vi "Ball-Detect(Vision).vi"(8 "error in (no error)":errorcluster, 11 "Image Size":T5=enum."320x240") -> ()   [LabVIEW 2019]
uses:
  <vilib>/Rock Robotics/WPI/Camera/WPI_CameraImageSize.ctl
  vision/Camera Types.ctl
  <vilib>/Rock Robotics/WPI/Camera/WPI_CameraWhite Balance Values.ctl
  <vilib>/Rock Robotics/WPI/Camera/WPI_CameraFrameRate.ctl
  Robot Global Data.vi
  <vilib>/Rock Robotics/WPI/Camera/WPI_CameraExposure Values.ctl
  <vilib>/vision/NI_Vision_Development_Module.lvlib
panel:
  out "Disqualified":i32
  in  "Details":bool
  out "Results":T1(array[cluster]) {"Normalized Center"."x" format="%#_2g"; "Normalized Center"."y" format="%#_2g"; "Overall Score" format="%#_2g"; "Distance (ft)" format="%#_3g"; "Area Score" format="%#_2g"; "Moment Score" format="%#_2g"; "Aspect Score" format="%#_2g"}
  in  "Size Limit %":dbl=0.1 min=0.0 max=100.0 step=0.01 format="%#_13g"
  in  "Color Mode":u16(ring)=2 items=["RGB", "HSL", "HSV", "HSI"]
  in  "Particle Count LImit":i32=5
  in  "Score Threshold %":dbl=75.0
  in  "Std Devs for Calibration":cluster{"H":dbl, "S":dbl, "V":dbl}={"H"=4.0, "S"=8.0, "V"=8.0}
  in  "Camera Type (for distance)":T2=enum."MS HD3000 square"
  in  "Annotate":bool=TRUE
  out "Qualified":i32
  in  "Color Range":T3={"Hue"={24.535868437582977, 35.591417062105585}, "Sat"={188.21428571428572, 255.0}, "Val"={118.39285714285714, 255.0}} {"Hue" scale=0.0..255.0 scale format="%#_3g"}
  out "Mask":T4(plugin-control)
  out "Original Image":T4(plugin-control)
  out "Instructions:":string="Connect a USB or IP camera to your roboRIO. If using a ring light and retroreflective tape, use Camera Settings outside the loop create a dark image with bright and colorful stripes. If used wihtout a ring light, brighten the images so that stripes are visible.\n\nLED Color can encoded as HSL or related color modes. Calibrate to the same color as the strips being reflected to the camera. Unlike the desktop example, this LED color must be set by hand. You can also put the calibration on the dashboard and send the LED Color to the RT code using Network Tables.\n\nThe Display buttons affects whether images are displayed on the panel. It takes quite a bit of CPU  to compress and transmit the images for display.\n\nAdjust Score Cutoff to make the code more or less picky. If the color is not very unique, you may need to increase the number of particles considered. The diagram uses a Size Limit to ignore colored things that are too small. You may need to adjust it if you are targetting from far away.\n\nResults give you the distance to the target, the center and box in a normalized (-1 to 1) and pixel coordinates.\n\nBe sure to read about setting camera exposure and brightness to help simplify your image and acquire color saturated images.\n\nThere are lots of comments on the diagram to explain the code."
  out "loop ms":u32
  # "Scores"
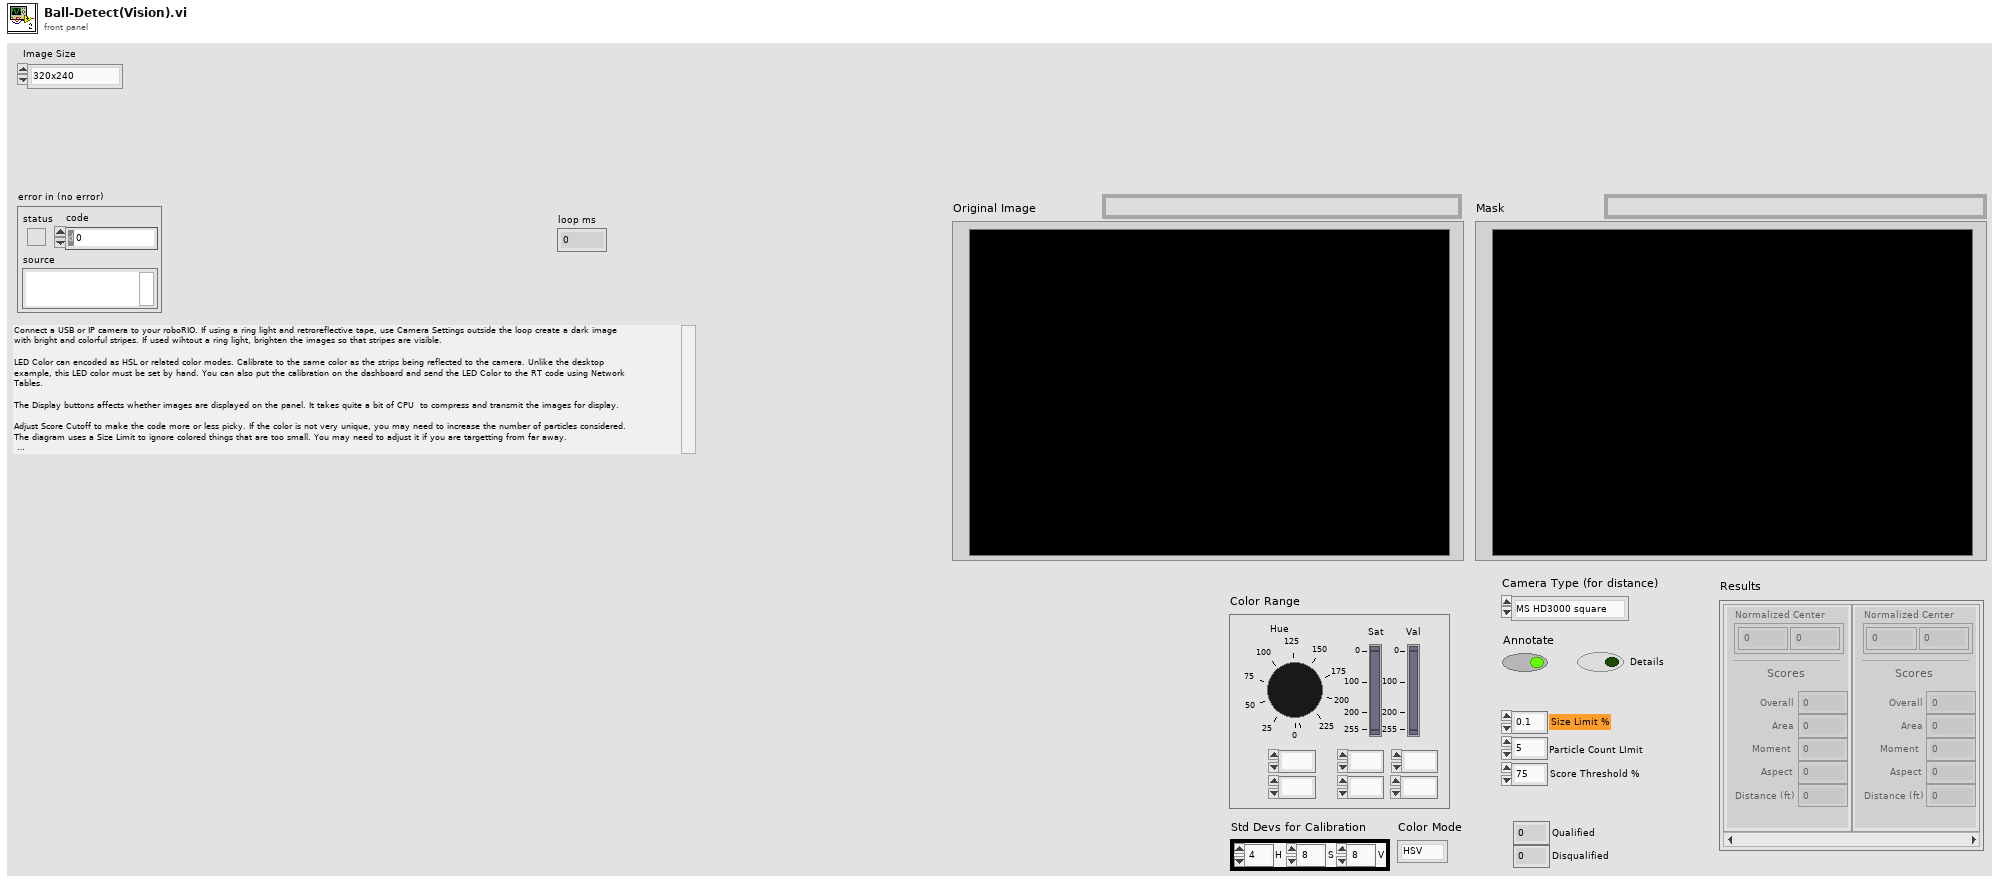
[diagram p1: front panel]
types:
  T1 = cluster{"diameter points":cluster{"first point":cluster{"x":dbl, "y":dbl}, "projected point":cluster{"x":dbl, "y":dbl}}, "Normalized Center":cluster{"x":dbl, "y":dbl}, "Overall Score":dbl, "Area Score":dbl, "Moment Score":dbl, "Aspect Score":dbl, "Distance (ft)":dbl, "Upper Goal":bool}[]
  T2 = typedef "Camera Types.ctl" = enum16{"206", "1011", "1013", "MS HD3000 square", "MS HD3000 640x480"}
  T3 = cluster{"Hue":cluster{dbl, dbl}, "Sat":cluster{dbl, dbl}, "Val":cluster{dbl, dbl}}
  T4 = typedef "IMAQ Image.ctl" = refnum<image>
  T5 = typedef "WPI_CameraImageSize.ctl" = enum16{"640x480", "320x240", "160x120", "Custom"}
  T6 = typedef "Particle Parameters" = i32
  T7 = typedef "WPI_CameraFrameRate.ctl" = u32
  T8 = typedef "WPI_CameraWhite Balance Values.ctl" = enum16{"Auto", "Fixed indoor", "Fixed outdoor 1", "Fixed outdoor 2", "Fixed fluorescent 1", "Fixed fluorescent 2", "Hold current", "Custom"}
  T9 = typedef "Image Type" = u32
  T10 = typedef "WPI_CameraDevRef.ctl" = cluster{"Camera Address":string, "CameraStatus":errorcluster}
  T11 = typedef "WPI_CameraExposure Values.ctl" = enum16{"Auto", "Flicker-free 50 Hz", "Flicker-free 60 Hz", "Hold current", "Custom"}
  T12 = cluster{cluster{dbl, dbl}, cluster{dbl, dbl}, cluster{dbl, dbl}}
  T13 = cluster{"remainder":i32, "size":bool, "count":bool}
  T14 = typedef "Target Fields.ctl" = cluster{"diameter points":cluster{"first point":cluster{"x":dbl, "y":dbl}, "projected point":cluster{"x":dbl, "y":dbl}}, "normalized center":cluster{"x":dbl, "y":dbl}, "Overall Score":dbl, "Area Score":dbl, "Moment Score":dbl, "Aspect Score":dbl, "Distance (ft)":dbl, "Upper Goal":bool}
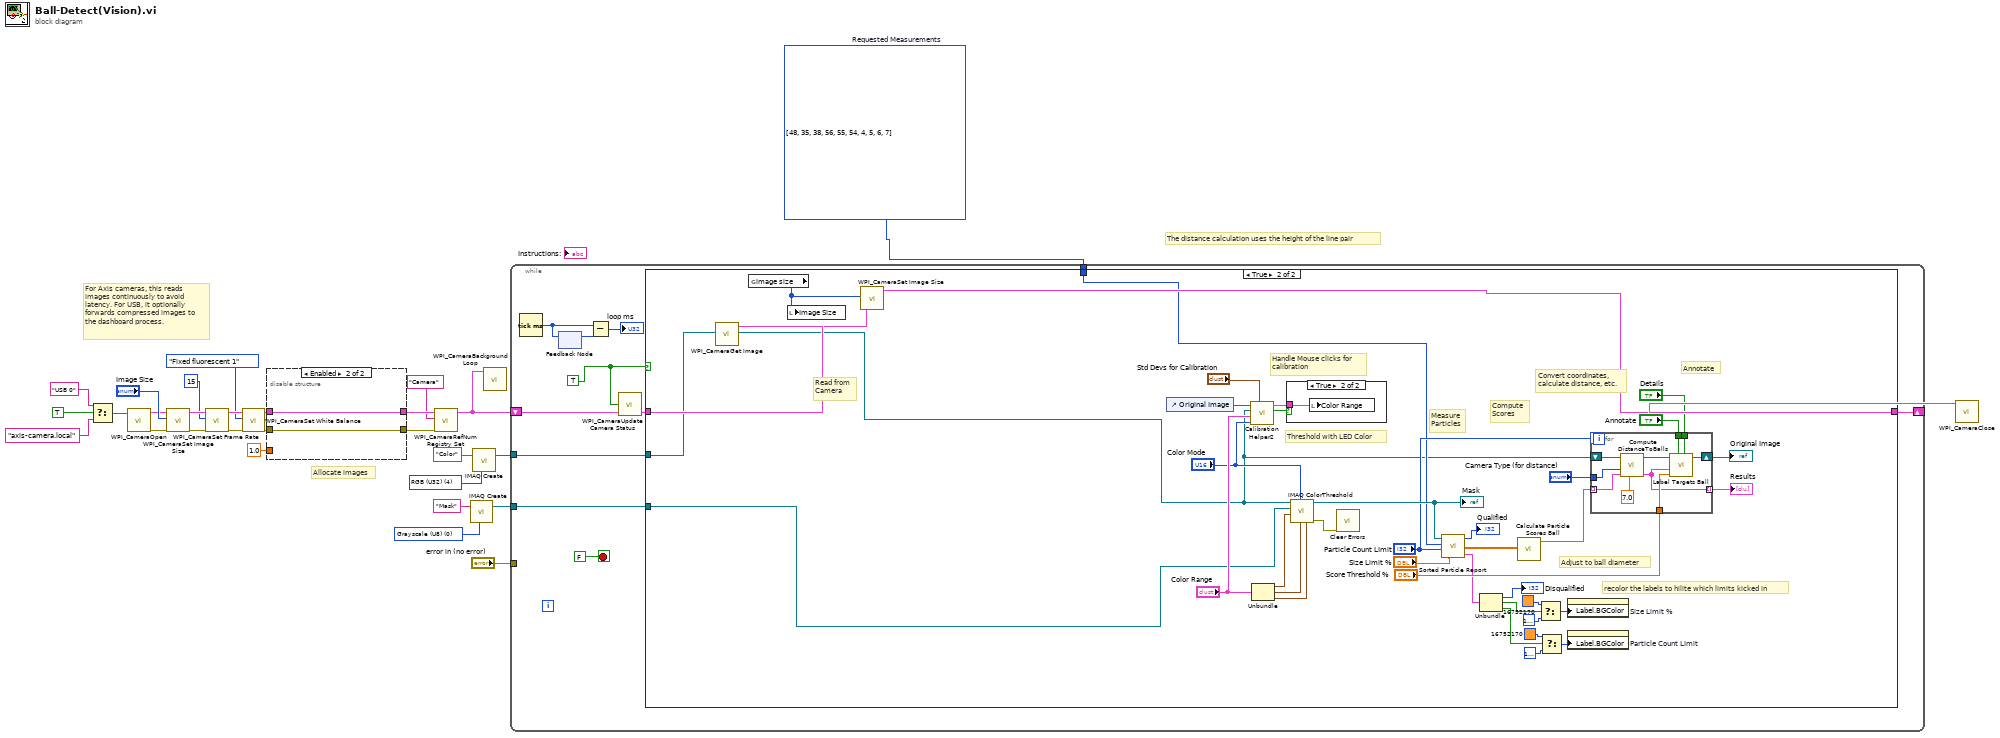
[diagram p0: block diagram]
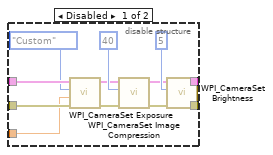
[diagram p2: hidden frame]
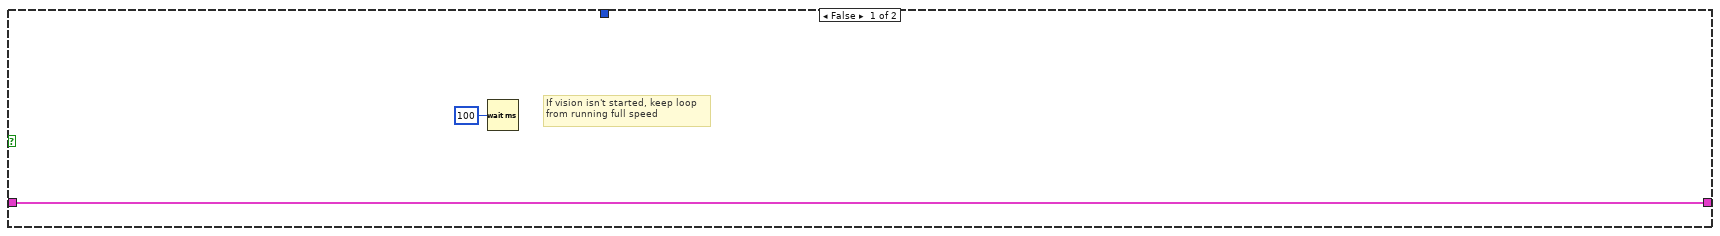
[diagram p3: hidden frame]
diagram:
  w1 = T6[] [48, 35, 38, 56, 55, 54, 4, 5, 6, 7] items=["Center of Mass X", "Center of Mass Y", "First Pixel X", "First Pixel Y", "Bounding Rect Left", "Bounding Rect Top", "Bounding Rect Right", "Bounding Rect Bottom", "Max Feret Diameter Start X", "Max Feret Diameter Start Y", "Max Feret Diameter End X", "Max Feret Diameter End Y", "Max Horiz. Segment Length Left", "Max Horiz. Segment Length Right", "Max Horiz. Segment Length Row", "-", "Bounding Rect Width", "Bounding Rect Height", "Bounding Rect Diagonal", "Perimeter", "Convex Hull Perimeter", "Holes' Perimeter", "Max Feret Diameter", "Equivalent Ellipse Major Axis", "Equivalent Ellipse Minor Axis", "Equivalent Ellipse Minor Axis (Feret)", "Equivalent Rect Long Side", "Equivalent Rect Short Side", "Equivalent Rect Diagonal", "Equivalent Rect Short Side (Feret)", "Average Horiz. Segment Length", "Average Vert. Segment Length", "Hydraulic Radius", "Waddel Disk Diameter", "-", "Area", "Holes' Area", "Particle & Holes' Area", "Convex Hull Area", "Image Area", "-", "Number of Holes", "Number of Horiz. Segments", "Number of Vert. Segments", "-", "Orientation", "Max Feret Diameter Orientation", "-", "% Area/Image Area", "% Area/(Particle & Holes' Area)", "Ratio of Equivalent Ellipse Axes", "Ratio of Equivalent Rect Sides", "-", "Elongation Factor", "Compactness Factor", "Heywood Circularity Factor", "Type Factor", "-", "Sum X", "Sum Y", "Sum XX", "Sum XY", "Sum YY", "Sum XXX", "Sum XXY", "Sum XYY", "Sum YYY", "-", "Moment of Inertia XX", "Moment of Inertia XY", "Moment of Inertia YY", "Moment of Inertia XXX", "Moment of Inertia XXY", "Moment of Inertia XYY", "Moment of Inertia YYY", "Norm. Moment of Inertia XX", "Norm. Moment of Inertia XY", "Norm. Moment of Inertia YY", "Norm. Moment of Inertia XXX", "Norm. Moment of Inertia XXY", "Norm. Moment of Inertia XYY", "Norm. Moment of Inertia YYY", "Hu Moment 1", "Hu Moment 2", "Hu Moment 3", "Hu Moment 4", "Hu Moment 5", "Hu Moment 6", "Hu Moment 7"]  # Requested Measurements
  w27 = T9 0 items=["Grayscale (U8)", "Grayscale (I16)", "Grayscale (SGL)", "Complex (CSG)", "RGB (U32)", "HSL (U32)", "RGB (U64)", "Grayscale (U16)"] ("Image Type")
  w28 = T9 4 items=["Grayscale (U8)", "Grayscale (I16)", "Grayscale (SGL)", "Complex (CSG)", "RGB (U32)", "HSL (U32)", "RGB (U64)", "Grayscale (U16)"] ("Image Type")
  # "For Axis cameras, this reads\nimages continuously to avoid\nlatency. For USB, it optionally\nforwards compressed images to\nthe dashboard process."
  # "The distance calculation uses the height of the line pair"
  # "Allocate images"
  n1 = Select(t="USB 0" ("format string"), s=TRUE ("dot notation? (F)"), f="axis-camera.local" ("format string")) -> (s? t:f=w6:string)
  n2 = call <vilib>:"WPI_CameraOpen.vi"("Camera Address"=w6) -> ("error out"=w15:errorcluster, "CameraDevRef"=w16:T10)  [unwired: 1 in, 8 out]
  n3 = call <vilib>:"WPI_CameraSet Image Size.vi"("error in (no error)"=w15, "Image Size"="Image Size", "CameraDevRef"=w16) -> ("error out"=w14:errorcluster, "CameraDevRef Out"=w17:T10)  [unwired: 1 in, 6 out]
  n4 = call <vilib>:"WPI_CameraSet Frame Rate.vi"("error in (no error)"=w14, "Frame Rate (fps)"=T7 15, "CameraDevRef"=w17) -> ("error out"=w13:errorcluster, "CameraDevRef Out"=w19:T10)  [unwired: 7 out]
  n5 = call <vilib>:"WPI_CameraSet White Balance.vi"("error in (no error)"=w13, "White Balance"=WPI_CameraWhite_Balance_Values."Fixed fluorescent 1", "CameraDevRef"=w19) -> ("error out"=w12:errorcluster, "CameraDevRef Out"=w18:T10)  [unwired: 1 in, 6 out]
  n6 = disable-structure shown="Enabled" {
    disable-tunnel: [w41 w43] -> w23
    disable-tunnel: w18 -> [w36 w43]
    disable-tunnel: w12 -> [w35 w42]
    disable-tunnel: [w32 w42] -> w11
    disable-tunnel: 1.0 ("Exposure (%)") -> [w30 _]
    frame Disabled {
      n7 = call <vilib>:"WPI_CameraSet Exposure.vi"("error in (no error)"=w35, "Exposure (%)"=w30, "Exposure"=WPI_CameraExposure_Values."Custom", "CameraDevRef"=w36) -> ("error out"=w34:errorcluster, "CameraDevRef Out"=w38:T10)  [unwired: 6 out]
      n8 = call <vilib>:"WPI_CameraSet Image Compression.vi"("error in (no error)"=w34, "Compression"=40, "CameraDevRef"=w38) -> ("error out"=w33:errorcluster, "CameraDevRef Out"=w37:T10)  [unwired: 7 out]
      n9 = call <vilib>:"WPI_CameraSet Brightness.vi"("error in (no error)"=w33, "Brightness"=5, "CameraDevRef"=w37) -> ("error out"=w32:errorcluster, "CameraDevRef Out"=w41:T10)  [unwired: 1 in, 6 out]
    }
    frame Enabled {
    }
  }
  n10 = call <vilib>:"WPI_CameraRefNum Registry Set.vi"("error in (no error)"=w11, "refnum name"="Camera", "CameraDevRef"=w23) -> ("CameraDevRef"=w5:T10)  [unwired: 1 in, 7 out]
  n11 = call "IMAQ Create"("Image Name"="Mask", "Image Type"=w27) -> ("New Image"=w25:T4)  [unwired: 2 in, 2 out]
  n12 = call "IMAQ Create"("Image Name"="Color", "Image Type"=w28) -> ("New Image"=w24:T4)  [unwired: 2 in, 2 out]
  n13 = call <vilib>:"WPI_CameraBackground Loop.vi"("CameraDevRef"=w5) -> ()  [unwired: 11 in]
  n14 = while {
    tunnel: w24 -> [w51]
    tunnel: w25 -> [w53]
    tunnel: w1 -> [w52]
    shift-right: [w50] -> w4
    shift-left: w5 -> [w49]
    tunnel: "error in (no error)" -> [_]
    stop <- FALSE stop-if-true
    w44 = TRUE
    n15 = Tick Count (ms)() -> (millisecond timer value=w46:u32)
    n16 = feedback #1() -> (w47:u32)  [unwired: 1 in]
    n17 = feedback-in #1(w46) -> ()
    n18 = Subtract(x=w46, y=w47) -> (x-y=→"loop ms":u32)
    n19 = call <vilib>:"WPI_CameraUpdate Camera Status.vi"("CameraDevRef In"=w49, "Enable Vision"=w44) -> ("CameraDevRef Out"=w48:T10)  [unwired: 3 in]
    n20 = case shown="True" w44 {
      tunnel: w53 -> [_ w60]
      tunnel: w52 -> [_ w59]
      tunnel: w48 -> [w56 w96]
      tunnel: w51 -> [_ w95]
      tunnel: [w56 w92] -> w50
      frame False {
        # "If vision isn't started, keep loop\nfrom running full speed"
        n21 = Wait (ms)(milliseconds to wait=u32 100) -> ()  [unwired: 1 out]
      }
      frame True {
        # "recolor the labels to hilite which limits kicked in"
        # "Adjust to ball diameter"
        # "Handle Mouse clicks for\ncalibration"
        # "Measure\nParticles"
        # "Convert coordinates,\ncalculate distance, etc."
        # "Annotate"
        # "Compute\nScores"
        # "Threshold with LED Color"
        # "Read from\nCamera"
        n22 = call <vilib>:"WPI_CameraGet Image.vi"("Image"=w95, "CameraDevRef"=w96) -> ("Image Out"=w58:T4, "CameraDevRef Out"=w94:T10)  [unwired: 7 in, 1 out]
        n23 = global read "Robot Global Data.vi" "image size"() -> (w93:T5)
        n24 = local write "Image Size"(w93) -> ()
        n25 = call <vilib>:"WPI_CameraSet Image Size.vi"("Image Size"=w93, "CameraDevRef"=w94) -> ("CameraDevRef Out"=w92:T10)  [unwired: 2 in, 7 out]
        n26 = control-ref of="Original Image"() -> (w86:refnum<vi>)
        n27 = call "Calibration Helper2.vi"("Std Devs"="Std Devs for Calibration", "Color Mode"="Color Mode", "Color Components"="Color Range", "Image"=w58, "Image Ctl Refnum"=w86) -> ("Changed"=w85:bool, "output color"=w84:T12)  [unwired: 5 in]
        n28 = Unbundle("Color Range") -> ("Hue"=w91:cluster{dbl, dbl}, "Sat"=w90:cluster{dbl, dbl}, "Val"=w89:cluster{dbl, dbl})
        n29 = case shown="True" w85 {
          tunnel: w84 -> [_ w97]
          frame False {
          }
          frame True {
            n30 = local write "Color Range"(w97) -> ()
          }
        }
        n31 = call "IMAQ ColorThreshold"("Blue or Luma or Val or Inten Range"=w89, "Green or Sat Range"=w90, "Color Mode"="Color Mode", "Red or Hue Range"=w91, "Image Dst"=w60, "Image Src"=w58) -> ("error out"=w75:errorcluster, "Image Dst Out"=w76:T4)  [unwired: 4 in]
        "Mask" <- w76
        n32 = call <vilib>:"Clear Errors.vi"("error in (no error)"=w75) -> ()  [unwired: 5 in, 2 out]
        n33 = call "Sorted Particle Report.vi"("Min Area Size %"="Size Limit %", "Particle Count Limit"="Particle Count LImit", "Pixel Measurements"=w59, "Image in"=w76) -> ("limits"=w71:T13, "Sorted Data"=w74:dbl[][], "Particles"=→"Qualified":i32)
        n34 = Unbundle(w71) -> ("remainder"=→"Disqualified":i32, "size"=w66:bool, "count"=w63:bool)
        n35 = call "Calculate Particle Scores Ball.vi"("Sorted Data"=w74) -> ("Scores"=w73:T14[])  [unwired: 10 in]
        n36 = Select(t=u32 16752170 ("Color"), s=w66, f=u32 16777216 ("Color")) -> (s? t:f=w65:u32)
        n37 = Select(t=u32 16752170 ("Color"), s=w63, f=u32 16777216 ("Color")) -> (s? t:f=w62:u32)
        n38 = property on="Size Limit %" class="DigNum (strict)"("Label.BGColor"=w65) -> ()  [unwired: 2 in, 2 out]
        n39 = property on="Particle Count LImit" class="DigNum (strict)"("Label.BGColor"=w62) -> ()  [unwired: 2 in, 2 out]
        n40 = for {
          N: "Particle Count LImit" -> [_]
          tunnel: w73 -> [w105] mode=indexing
          tunnel: "Camera Type (for distance)" -> [w102]
          tunnel: "Annotate" -> [w99]
          shift-right: [w107] -> w78
          shift-left: w58 -> [w101]
          tunnel: "Score Threshold %" -> [w106]
          tunnel: [w104] -> w57 mode=indexing
          tunnel: "Details" -> [w98]
          n41 = call "Compute DistanceToBalls.vi"("Target Width (in)"=7.0, "results"=w105, "Camera Type"=w102, "Image Src"=w101) -> ("results out"=w104:T14, "Image Dst Out"=w103:T4)  [unwired: 6 in]
          n42 = call "Label Targets Ball.vi"("Details"=w98, "Annotate"=w99, "Score Threshold"=w106, "results"=w104, "Image in"=w103) -> ("Image out"=w107:T4)  [unwired: 6 in]
        }
        "Original Image" <- w78
        "Results" <- w57
      }
    }
  }
  n43 = call <vilib>:"WPI_CameraClose.vi"("CameraDevRef"=w4) -> ()  [unwired: 1 in, 10 out]
